vi "Find_Place_in_Stat_Tree_for_Dot-2.vi"(4 "[IN] Closing gaps":i32 min=1, 5 "[IN] dR min":dbl, 6 "# frame = \nindex of dot":i32, 7 "Y":dbl, 8 "X":dbl, 9 "[IN] Stationary Dots":T1(array[cluster])) -> (1 "Potential unmoving \ndot is allocated":bool, 3 "[OUT] Stationary Dots \nwith Additional Points":T1(array[cluster]))   [LabVIEW 2013]
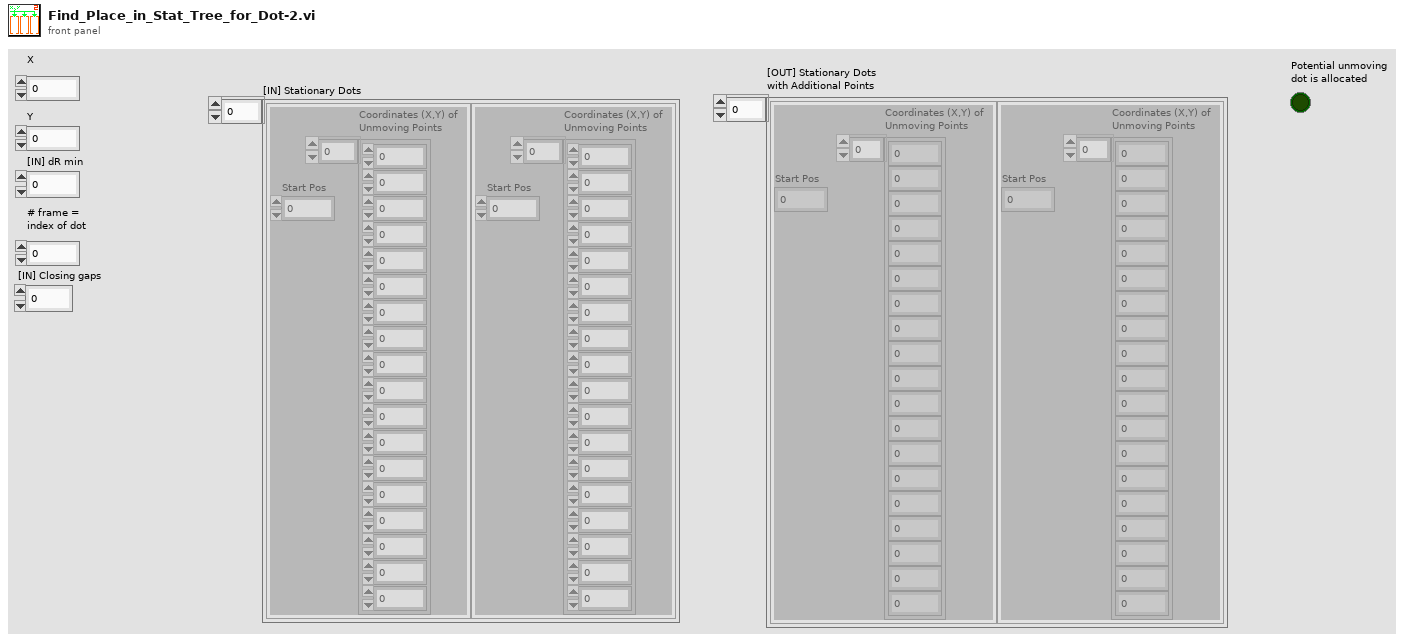
[diagram p1: front panel]
types:
  T1 = cluster{"Coordinates (X,Y) of\nUnmoving Points":dbl[], "Start Pos":i32}[]
  T2 = cluster{"Coordinates (X,Y) of\nUnmoving Points":dbl[], "Start Pos":i32}
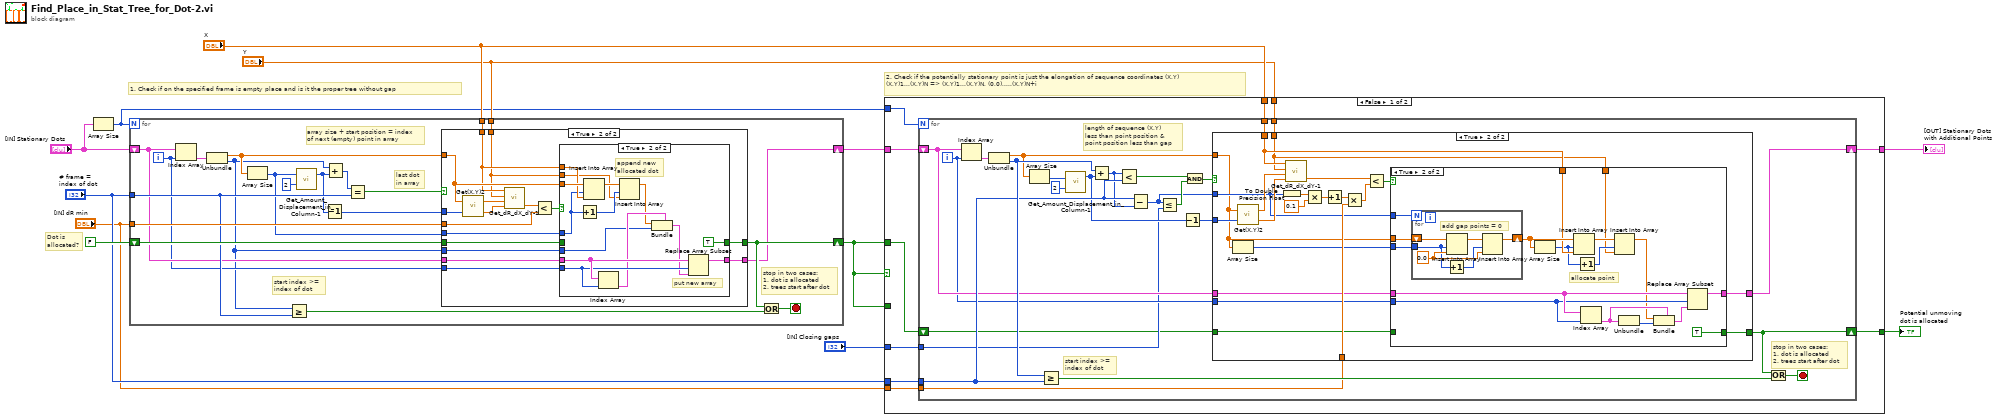
[diagram p0: block diagram]
diagram:
  # "2. Check if the potentially stationary point is just the elongation of sequence coordinates (X,Y)\n(X,Y)1...(X,Y)N => (X,Y)1...(X,Y)N, (0,0),....(X,Y)N+i"
  # "Dot is \nallocated?"
  # "1. Check if on the specified frame is empty place and is it the proper tree without gap"
  n1 = Array Size(array="[IN] Stationary Dots") -> (size(s)=w3:i32)
  n2 = for {
    N: w3 -> [_]
    tunnel: "# frame = \nindex of dot" -> [w23]
    tunnel: "X" -> [w32]
    tunnel: "Y" -> [w31]
    tunnel: "[IN] dR min" -> [w30]
    shift-right: [w28] -> w2
    shift-left: FALSE -> [w29]
    shift-right: [w14] -> w4
    shift-left: "[IN] Stationary Dots" -> [w17]
    i -> [w16]
    stop <- w27 stop-if-true
    # "last dot \nin array"
    # "array size + start position = index \nof next (empty) point in array"
    # "start index >= \nindex of dot"
    # "stop in two cases: \n1. dot is allocated\n2. trees start after dot"
    n3 = Index Array(array=w17, index=w16) -> (element=w18:T2)
    n4 = Unbundle(w18) -> ("Coordinates (X,Y) of\nUnmoving Points"=w26:dbl[], "Start Pos"=w15:i32)
    n5 = Array Size(array=w26) -> (size(s)=w19:i32)
    n6 = Greater Or Equal?(x=w15, y=w23) -> (x >= y?=w13:bool)
    n7 = call "Get_Amount_Displacement_in_Column-1.vi"("multiplier"=2 ("y"), "# Rows"=w19) -> ("Displ amount"=w21:i32)  [unwired: 1 out]
    n8 = Decrement(x=w21) -> (x-1=w20:i32)
    n9 = Add(x=w15, y=w21) -> (x+y=w24:i32)
    n10 = Equal?(x=w24, y=w23) -> (x = y?=w22:bool)
    n11 = case shown="True" w22 {
      tunnel: w26 -> [_ w45]
      tunnel: w32 -> [_ w44]
      tunnel: w31 -> [_ w43]
      tunnel: w30 -> [_ w47]
      tunnel: w29 -> [w34 w42]
      tunnel: [w34 w41] -> w28
      tunnel: w20 -> [_ w40]
      tunnel: w19 -> [_ w39]
      tunnel: w17 -> [w33 w38]
      tunnel: w16 -> [_ w37]
      tunnel: w15 -> [_ w36]
      tunnel: [w33 w35] -> w14
      frame False {
      }
      frame True {
        n12 = call "Get(X,Y)2.vi"("[IN] index of (X,Y)"=w40, "[IN] Array coordi\nnates (X,Y) in Frame"=w45) -> ("[OUT] Y"=w49:dbl, "[OUT] X"=w50:dbl)
        n13 = call "Get_dR_dX_dY-1.vi"("Y2"=w49, "X2"=w50, "Y1"=w43, "X1"=w44) -> ("dR"=w48:dbl)  [unwired: 2 out]
        n14 = Less?(x=w48, y=w47) -> (x < y?=w46:bool)
        n15 = case shown="True" w46 {
          tunnel: w45 -> [_ w65]
          tunnel: w44 -> [_ w64]
          tunnel: w43 -> [_ w60]
          tunnel: w42 -> [w52 _]
          tunnel: [w52 TRUE] -> w41
          tunnel: w39 -> [_ w63]
          tunnel: w38 -> [w51 w59]
          tunnel: w37 -> [_ w58]
          tunnel: w36 -> [_ w55]
          tunnel: [w51 w53] -> w35
          frame False {
          }
          frame True {
            # "put new array"
            # "append new\nallocated dot"
            n16 = Increment(x=w63) -> (x+1=w61:i32)
            n17 = Insert Into Array(array=w65, index=w63, new element=w64) -> (w62:dbl[])
            n18 = Index Array(array=w59, index=w58) -> (element=w57:T2)
            n19 = Insert Into Array(array=w62, index=w61, new element=w60) -> (w56:dbl[])
            n20 = Bundle(cluster=w57, "Coordinates (X,Y) of\nUnmoving Points"=w56, "Start Pos"=w55) -> (w54:T2)
            n21 = Replace Array Subset(array=w59, new element=w54, index=w58) -> (w53:T1)
          }
        }
      }
    }
    n22 = Or(x=w28, y=w13) -> (x .or. y?=w27:bool)
  }
  n23 = case shown="False" w2 {
    tunnel: "# frame = \nindex of dot" -> [w72 _]
    tunnel: w2 -> [_ w150]
    tunnel: "[IN] Closing gaps" -> [w68 _]
    tunnel: "X" -> [w71 _]
    tunnel: "Y" -> [w70 _]
    tunnel: "[IN] dR min" -> [w75 _]
    tunnel: [w69 w150] -> w6
    tunnel: w4 -> [w76 w149]
    tunnel: w3 -> [w74 _]
    tunnel: w2 -> [w73 _]
    tunnel: [w67 w149] -> w1
    frame False {
      n24 = for {
        N: w74 -> [_]
        tunnel: w75 -> [w86]
        shift-right: [w78] -> w69
        shift-left: w73 -> [w77]
        shift-right: [w79] -> w67
        shift-left: w76 -> [w82]
        tunnel: w72 -> [w94]
        tunnel: w71 -> [w88]
        tunnel: w70 -> [w87]
        tunnel: w68 -> [w80]
        i -> [w81]
        stop <- w100 stop-if-true
        # "length of sequence (X,Y)\nless than point position &\npoint position less than gap"
        # "start index >= \nindex of dot"
        # "stop in two cases: \n1. dot is allocated\n2. trees start after dot"
        n25 = Index Array(array=w82, index=w81) -> (element=w99:T2)
        n26 = Unbundle(w99) -> ("Coordinates (X,Y) of\nUnmoving Points"=w89:dbl[], "Start Pos"=w95:i32)
        n27 = Array Size(array=w89) -> (size(s)=w96:i32)
        n28 = Greater Or Equal?(x=w95, y=w94) -> (x >= y?=w98:bool)
        n29 = call "Get_Amount_Displacement_in_Column-1.vi"("multiplier"=2 ("y"), "# Rows"=w96) -> ("Displ amount"=w85:i32)  [unwired: 1 out]
        n30 = Add(x=w95, y=w85) -> (x+y=w83:i32)
        n31 = Less?(x=w83, y=w94) -> (x < y?=w92:bool)
        n32 = Subtract(x=w94, y=w83) -> (x-y=w90:i32)
        n33 = Less Or Equal?(x=w90, y=w80) -> (x <= y?=w93:bool)
        n34 = Decrement(x=w85) -> (x-1=w84:i32)
        n35 = And(x=w92, y=w93) -> (x .and. y?=w91:bool)
        n36 = case shown="True" w91 {
          tunnel: w90 -> [_ w112]
          tunnel: w89 -> [_ w111]
          tunnel: w84 -> [_ w123]
          tunnel: w88 -> [_ w109]
          tunnel: w87 -> [_ w108]
          tunnel: w86 -> [_ w115]
          tunnel: [w101 w107] -> w78
          tunnel: w82 -> [w102 w106]
          tunnel: w81 -> [_ w105]
          tunnel: [w102 w104] -> w79
          tunnel: w77 -> [w101 w103]
          frame False {
          }
          frame True {
            n37 = Array Size(array=w111) -> (size(s)=w110:i32)
            n38 = call "Get(X,Y)2.vi"("[IN] index of (X,Y)"=w123, "[IN] Array coordi\nnates (X,Y) in Frame"=w111) -> ("[OUT] Y"=w121:dbl, "[OUT] X"=w122:dbl)
            n39 = To Double Precision Float(number=w112) -> (double precision float=w119:dbl)
            n40 = call "Get_dR_dX_dY-1.vi"("Y2"=w121, "X2"=w122, "Y1"=w108, "X1"=w109) -> ("dR"=w120:dbl)  [unwired: 2 out]
            n41 = Multiply(x=w119, y=0.1) -> (x*y=w117:dbl)
            n42 = Increment(x=w117) -> (x+1=w116:dbl)
            n43 = Multiply(x=w116, y=w115) -> (x*y=w114:dbl)
            n44 = Less?(x=w120, y=w114) -> (x < y?=w113:bool)
            n45 = case shown="True" w113 {
              tunnel: w112 -> [_ w142]
              tunnel: w111 -> [_ w141]
              tunnel: w110 -> [_ w140]
              tunnel: w109 -> [_ w138]
              tunnel: w108 -> [_ w134]
              tunnel: [w124 TRUE] -> w107
              tunnel: w106 -> [w125 w132]
              tunnel: w105 -> [_ w131]
              tunnel: [w125 w126] -> w104
              tunnel: w103 -> [w124 _]
              frame False {
              }
              frame True {
                # "allocate point"
                n46 = for {
                  N: w142 -> [_]
                  shift-right: [w143] -> w139
                  shift-left: w141 -> [w148]
                  tunnel: w140 -> [w145]
                  w146 = 0.0 ("new element/subarray")
                  # "add gap points = 0"
                  n47 = Increment(x=w145) -> (x+1=w144:i32)
                  n48 = Insert Into Array(array=w148, index=w145, new element=w146) -> (w147:dbl[])
                  n49 = Insert Into Array(array=w147, index=w144, new element=w146) -> (w143:dbl[])
                }
                n50 = Array Size(array=w139) -> (size(s)=w137:i32)
                n51 = Insert Into Array(array=w139, index=w137, new element=w138) -> (w135:dbl[])
                n52 = Increment(x=w137) -> (x+1=w136:i32)
                n53 = Index Array(array=w132, index=w131) -> (element=w130:T2)
                n54 = Insert Into Array(array=w135, index=w136, new element=w134) -> (w128:dbl[])
                n55 = Unbundle(w130) -> ("Start Pos"=w129:i32)  [unwired: 1 out]
                n56 = Bundle(cluster=w130, "Coordinates (X,Y) of\nUnmoving Points"=w128, "Start Pos"=w129) -> (w127:T2)
                n57 = Replace Array Subset(array=w132, new element=w127, index=w131) -> (w126:T1)
              }
            }
          }
        }
        n58 = Or(x=w78, y=w98) -> (x .or. y?=w100:bool)
      }
    }
    frame True {
    }
  }
  "Potential unmoving \ndot is allocated" <- w6
  "[OUT] Stationary Dots \nwith Additional Points" <- w1
